vi "IVCurvePulsed.vi"(9 "Source Measure Unit Channel (0: Channel A)":i32, 10 "Waveform":waveform(dbl), 11 "VISA Refnum in":refnum<visa-resource-name>) -> (1 "appended array":dbl[][](array[numeric]), 3 "Cluster":cluster{"Y":dbl[], "Current (A)":dbl[]})   [LabVIEW 2020]
uses:
  <vilib>/Analysis/6fits.llb/Curve Fitting Criteria.ctl
  <vilib>/Utility/file.llb/Write Delimited Spreadsheet (DBL).vi
  Keithley 2600 Series/Keithley 2600 Series.lvlib
  <vilib>/Analysis/NI_AALPro.lvlib
panel:
  out "XY Graph 2":cluster{dbl[], dbl[]}[](graph)
  out "Fit":dbl[](array[numeric])
  out "error out 2":errorcluster
  out "Waveform Graph":waveform(dbl)(graph)
  out "XY Graph":T1(graph)
  out "error out":errorcluster
  in  "Source Code":string="-- The local functions are scoped at the project level, so that we can keep\n-- track of the reading buffers throughout the test.\nreset()\nsmua.reset()\nlocal systemNodes = {}\nlocal systemSmus = {}\nlocal systemSmuReadingBufferIndexes = {}\nlocal appendMode = 1\n\nlocal gOverrunDetected = false\n--==========================================================================\n-- This function tests for overruns in any of the system smus' trigger models.\n-- It returns an error to the application that will be displayed in a\n-- dialog box if an overrun occurs.\n--==========================================================================\nlocal _Overruncheck = function()\n    --==========================================================================\n    -- This function test the results of the value in the smu's trigger overrun\n    -- status register. -- It returns an error if an overrun occurs.\n    --\n    -- parameter   overrun     A bit pattern that contains the smu trigger overrun\n    --                         status register result\n    --==========================================================================\n    local TestOverrunBits = function(overrun, selNode, whichSmu)\n        local whichNode = [[localnode.]]\n        if (selNode.tsplink.node ~= localnode.tsplink.node) then\n            whichNode = [[node[]] .. selNode.tsplink.node .. [[].]]\n        end\n        whichNode = whichNode .. whichSmu .. [[ (]] .. selNode.model .. [[)]]\n        if (bit.test(overrun, 2)) then\n            gOverrunDetected = true\n            return(\"arm overrun on \" .. whichNode .. \"{eol}\")\n        elseif (bit.test(overrun, 3)) then\n            gOverrunDetected = true\n            return(\"source overrun on \" .. whichNode .. \"{eol}\")\n        elseif (bit.test(overrun, 4)) then\n            gOverrunDetected = true\n            return(\"measure overrun on \" .. whichNode .. \"{eol}\")\n        elseif (bit.test(overrun, 5)) then\n            gOverrunDetected = true\n        return(\"end pulse overrun on \" .. whichNode .. \"{eol}\")\n    else\n        return(\"\")\n    end\nend\n\n-- Report an overrun error only once.\nif(gOverrunDetected == false) then\n    local allSmusInOverrun = [[]]\n    \n    for i, selNode in ipairs(systemNodes) do\n        for j, selSmu in ipairs(systemSmus[i]) do\n            if(j == 1) then\n                local overrun = selNode.status.operation.instrument.smua.trigger_overrun.event\n                if (overrun > 0) then\n                    allSmusInOverrun = allSmusInOverrun .. TestOverrunBits(overrun, selNode, [[smua]])\n                end\n            elseif(j == 2) then\n                local overrun = selNode.status.operation.instrument.smub.trigger_overrun.event\n                if (overrun > 0) then\n                    allSmusInOverrun = allSmusInOverrun .. TestOverrunBits(overrun, selNode, [[smub]])\n                end\n            end\n        end\n    end\n    \n    if (gOverrunDetected == true) then\n        print(\"[{error}]Script stopped due to:{eol}\" .. allSmusInOverrun)\n    end\nend\nend\n\nlocal gComplianceDetected = false\n--==========================================================================\n-- Checks smus for voltage or current compliance.\n-- If a compliance event occurs, the message dialog box is presented to the\n-- user.\n--==========================================================================\nlocal _ComplianceCheck = function()\n    -- Report a compliance error only once.\n    if(gComplianceDetected == false) then\n        local allSmusInCompliance = [[]]\n        \n        for i, selNode in ipairs(systemNodes) do\n            for j, selSmu in ipairs(systemSmus[i]) do\n                local compDetect = selNode.status.measurement.instrument.event\n                if(compDetect > 0) then\n                    -- Compose and show error message\n                    local whichNode = [[localnode.]]\n                    if (selNode.tsplink.node ~= localnode.tsplink.node) then\n                        whichNode = [[node[]] .. selNode.tsplink.node .. [[].]]\n                    end\n                    local whichSmu = [[]]\n                    if(compDetect == 2) then\n                        whichSmu = whichNode .. [[smua]]\n                    elseif (compDetect == 4) then\n                        whichSmu = whichNode .. [[smub]]\n                    elseif (compDetect == 6) then\n                        whichSmu = whichNode .. [[smua and ]] .. whichNode .. [[smub]]\n                    end\n                    whichSmu = whichSmu .. [[ (]] .. selNode.model .. [[){eol}]]\n                    allSmusInCompliance = allSmusInCompliance .. whichSmu\n                    \n                    -- Set gComplianceDetected so we don't report the error again.\n                    gComplianceDetected = true\n                end\n            end\n        end\n        \n        if (gComplianceDetected == true) then\n            print(\"[{info}]Compliance detected on:{eol}\" .. allSmusInCompliance ..\n            \"{eol}Click the Advanced button and check the Source Limit setting.\")\n        end\n    end\nend\n\nlocal gTestAborted = false\n--==========================================================================\n-- This function waits up to a specified period for the sweeps to complete.\n-- If the delay parameter is -1, then the timeout is infinite. It returns true\n-- if all sweeping actions are complete. Otherwise, the return value is false.\n-- Note: If gTestAborted is true, this function returns false immediately.\n--\n-- parameter  interval     Maximum time to wait (in seconds).\n--==========================================================================\nlocal _WaitForComplete = function(interval)\n    local pollInterval = 0.1\n    \n    --==========================================================================\n    -- Checks the system smus for any that are still sweeping.\n    --==========================================================================\n    local IsSweepingComplete = function()\n        for i, selNode in ipairs(systemNodes) do\n            for j, selSmu in ipairs(systemSmus[i]) do\n                if (j == 1) then\n                    local statcond = selNode.status.operation.instrument.smua.condition\n                    if (bit.test(statcond,4)) then\n                        return false\n                    end\n                elseif (j == 2) then\n                    local statcond = selNode.status.operation.instrument.smub.condition\n                    if (bit.test(statcond,4)) then\n                        return false\n                    end\n                end\n            end\n        end\n        \n        return true\n    end\n    \n    local notimeout = false\n    if (interval < 0) then\n        notimeout = true\n        interval = 1\n    end\n    \n    while(interval > 0) do\n        -- Check the abort flag\n        if (gTestAborted == true) then\n            return false\n        end\n        \n        -- Check for errors\n        if (errorqueue.count > 0) then\n            return false\n        end\n        \n        -- Check for overruns and compliance\n        _Overruncheck()\n        _ComplianceCheck()\n        \n        if (IsSweepingComplete() == true) then\n            return true\n        end\n        \n        delay(pollInterval)\n        \n        if (notimeout == false) then\n            interval = interval - pollInterval\n        end\n    end\n    \n    if (IsSweepingComplete() == true) then\n        return true\n    end\n    \n    return false\nend\n----------------------------------------------------------------------------\n-- START OF INITIALIZE SEGMENT ... do not modify this section\n----------------------------------------------------------------------------\n--==========================================================================\n-- This function prepares the test for execution. \n-- It first verifies that current setup matches project's setup. \n-- Then, it initializes members used to keep track of reading buffer storage.\n--==========================================================================\nfunction _Initialize()\n    local maxNodes = 64   -- Maximum possible nodes in TSP link system.\n    \n    local projectSetup = {{localnode,[[2636A]],[[2.2.1]]}} -- Instrument configuration for the project.\n    local currentSetup = {} -- Current instrument configuration.\n    \n    local errorTag = \"[{error}]\"\n    local errorMessage = {[[Instrument in project configuration not found.]], [[Instrument configuration at does not match.]]}\n    local errorNo = 0\n    \n    --==========================================================================\n    -- Configures the status model to detect voltage or current compliance.\n    --==========================================================================\n    local ConfigStatusModel = function()\n        for i, selNode in ipairs(systemNodes) do\n            selNode.status.reset()\n            for j, selSmu in ipairs(systemSmus[i]) do\n                -- The selSmu.source.compliance call will force an update\n                -- the condition register of the measurement.instrument.smuX to\n                -- update\n                local dum = selSmu.source.compliance\n                if(j == 1) then\n                    -- Clear the measurement.instrument.smua event register by reading its value\n                    dum = selNode.status.measurement.instrument.smua.event\n                    -- Now configure the status model to detect voltage or current compliance\n                    selNode.status.measurement.instrument.smua.enable = 3\n                    selNode.status.measurement.instrument.smua.ptr = 3\n                    selNode.status.measurement.instrument.enable = 6\n                    selNode.status.measurement.instrument.ptr = 6\n                elseif(j == 2) then\n                    -- Clear the measurement.instrument.smub event register by reading its value\n                    dum = selNode.status.measurement.instrument.smub.event\n                    -- Now configure the status model to detect voltage or current compliance\n                    selNode.status.measurement.instrument.smub.enable = 3\n                    selNode.status.measurement.instrument.smub.ptr = 3\n                end\n            end\n        end\n    end\n    \n    --==========================================================================\n    -- Determines the current system configuration.\n    --==========================================================================\n    local GetSetup = function ()\n        local masterNode = tsplink.node\n        \n        systemSmus = {}\n        systemNodes = {}\n        systemNodes[1] = node[masterNode]\n        \n        currentSetup[1] = {}\n        currentSetup[1][1] = node[masterNode]\n        currentSetup[1][2] = node[masterNode].model\n        currentSetup[1][3] = node[masterNode].revision\n        \n        systemSmus[1] = {}\n        systemSmus[1][1] = node[masterNode].smua\n        \n        if(node[masterNode].smub ~= nil) then\n            systemSmus[1][2] = node[masterNode].smub\n        end\n        \n        local j = 2\n        for i = 1, maxNodes do\n            if((tsplink.node ~= i) and (node[i] ~= nil)) then\n                systemNodes[j] = node[i]\n                currentSetup[j] = {}\n                currentSetup[j][1] = node[i]\n                currentSetup[j][2] = node[i].model\n                currentSetup[j][3] = node[i].revision\n                \n                systemSmus[j] = {}\n                systemSmus[j][1] = node[i].smua\n                \n                if(node[i].smub ~= nil) then\n                    systemSmus[j][2] = node[i].smub\n                end\n                j = j +1\n            end\n        end\n    end\n    \n    GetSetup()\n    \n    -- Check the project setup versus the configuration setup.\n    -- If there is a difference, report an error.\n    local numpInstruments = table.getn(projectSetup)\n    local numcInstruments = table.getn(currentSetup)\n    \n    for i=1, numpInstruments do\n        local pfields = table.getn(projectSetup[i])\n        \n        errorNo = 1\n        for j=1,numcInstruments do\n            -- Compare nodes.\n            if(projectSetup[i][1] ==  currentSetup[j][1]) then\n                errorNo = 0\n                \n                for k=2, pfields do\n                    if(projectSetup[i][k] ~= currentSetup[j][k]) then\n                        errorNo = 2\n                    end\n                end\n                break\n            end\n        end\n        \n        if (errorNo > 0) then\n            break\n        end\n    end\n    \n    if (errorNo > 0) then\n        error(errorMessage[errorNo])\n        print(errorTag .. errorMessage[errorNo])\n    end\n    \n    --==========================================================================\n    -- Initializes all system readings buffers by clearing and setting them to\n    -- append mode. An array, sysSmuReadingBufferIndexes, is used to keep track of the\n    -- data stored to each of the reading buffers.\n    --==========================================================================\n    local InitalizeReadingBuffers = function()\n        systemSmuReadingBufferIndexes = {}\n        for i, selNode in ipairs(systemSmus) do\n            systemSmuReadingBufferIndexes[i] = {}\n            \n            for j, selSmu in ipairs(selNode) do\n                -- Create an array for the smu.\n                systemSmuReadingBufferIndexes[i][j] = {}\n                \n                local snvBuffers =  {selSmu.nvbuffer1, selSmu.nvbuffer2}\n                for k, selBuffer in ipairs(snvBuffers) do\n                    -- Create an array for nvbuffers 1 and 2.\n                    systemSmuReadingBufferIndexes[i][j][k] = {}\n                    \n                    local sysSmuReadingBufferIndexes = systemSmuReadingBufferIndexes[i][j][k]\n                    sysSmuReadingBufferIndexes[\"start\"] = 0\n                    sysSmuReadingBufferIndexes[\"stop\"] = 0\n                    \n                    selBuffer.clear()\n                    selBuffer.appendmode = 1\n                    selBuffer.collecttimestamps = 1\n                    selBuffer.collectsourcevalues = 1\n                    selBuffer.timestampresolution = 1e-6\n                    if (selBuffer.fillmode ~= nil) then\n                        selBuffer.fillmode = selSmu.FILL_ONCE\n                    end\n                end\n                \n            end\n        end\n    end\n    \n    InitalizeReadingBuffers()\n    ConfigStatusModel()\nend\n----------------------------------------------------------------------------\n-- END OF INITIALIZE SEGMENT ... do not modify code after this point\n----------------------------------------------------------------------------\n\n----------------------------------------------------------------------------\n-- START OF SWEEP SEGMENT ... do not modify this section\n----------------------------------------------------------------------------\n--==========================================================================\n-- Configures a sweeping test.\n-- (This represents a Sweep segment of the script.  Click on the Sweep tab to customize it.)\n--==========================================================================\nfunction _Sweep()\n    local highSpeedSampling = false\n    local errorTag = \"[{error}]\"\n    local biasIndex = 1\n    local stepIndex = 2\n    local sweepIndex = 3\n    local numLevels = 3\n    local nvBuffersUsed = {1,1,1}\n    -- local alias for SMUs\n    local sweep1 = localnode.smua -- is a 2636A\n    -- \"NoStepFixed\" configuration (autorange enabled = false,  #step channels = 0):\n    -- This function configures any number of sweeping smus with no stepping smus.\n    -- It supports sweeps with autorange off and pulse mode.\n    local testSmus = {\n        {{}},  -- Bias\n        {{}},  -- Step\n        {{ localnode.smua }},  -- Sweep\n    }\n    \n    local testNodes = {\n        {},  -- Bias\n        {},  -- Step\n        {localnode}  -- Sweep\n    }\n    \n    local sweepPulseModes ={{ false }}\n    \n    local timePoint = 0.1\n    local pulseWidth = 99.0000009537E-3\n    local measurePointTime = 16.7266666667E-3\n    \n    local numberOfSteps  =  1\n    local numberOfSweeps = #NumPoints\n    \n    local nplc = 1\n    local lineFrequency = 60\n    \n    local numNodes = table.getn(testNodes[sweepIndex])\n    local numMasterSmus = table.getn(testSmus[sweepIndex][1])\n    local masterNode = testNodes[sweepIndex][1]\n    local masterSweepSmu = testSmus[sweepIndex][1][1]\n    \n    local t1Timer = masterNode.trigger.timer[1]    -- t1Timer is for sweep time per point\n    local t2Timer = masterNode.trigger.timer[2]    -- t2Timer is for sweep pulse width\n    local t3Timer = masterNode.trigger.timer[3]    -- t3Timer is for a 1ms initial delay\n    \n    local masterTspLine1 = masterNode.tsplink.trigger[1]    -- for source stimulus\n    local masterTspLine2 = masterNode.tsplink.trigger[2]    -- for endpulse stimulus\n    \n    --==========================================================================\n    -- This function checks for errors or conflicts in the test settings (timing, ranges, etc.)\n    --==========================================================================\n    local CheckSettings = function()\n        local measureDelay = timePoint - measurePointTime\n        \n        local errorMsg = nil\n        \n        -- Valid timing paramaters\n        -- None of these errors should appear to the user.\n        if (masterSweepSmu == nil) then\n            errorMsg =  [[Must have at least one sweeping smu.]]\n        elseif (timePoint <= 0) then\n            errorMsg = [[timePoint <= 0]]\n        elseif (pulseWidth <= 0) then\n            errorMsg = [[pulseWidth <= 0]]\n        elseif (pulseWidth > timePoint) then\n            errorMsg = [[pulseWidth > timePoint]]\n        elseif (measureDelay < 0) then\n            errorMsg = [[timePoint too small, <= measurePointTime]]\n        end\n        \n        if (errorMsg ~= nil) then\n            print(errorTag.. errorMsg)\n            error(errorMsg)\n        end\n    end\n    \n    --==========================================================================\n    -- This function configures the trigger line interaction between the smus.\n    --==========================================================================\n    local ConfigureTriggerLines = function()\n        --==========================================================================\n        -- This function configures the timers that are used in the test.\n        --==========================================================================\n        local ConfigureSweepTimers = function()\n            -- t3Timer provides a 1ms initial delay following the masterSweepSmu's armed event ID.\n            -- This is to ensure that masterSweepSmu is fully ready for the first source stimulus.\n            t3Timer.stimulus = masterSweepSmu.trigger.ARMED_EVENT_ID\n            t3Timer.passthrough = false\n            t3Timer.delay = 1.0e-3\n            t3Timer.count = 1\n            \n            if (numberOfSweeps > 1) then\n                t1Timer.stimulus = t3Timer.EVENT_ID\n                t1Timer.passthrough = true\n                t1Timer.delay = timePoint\n                t1Timer.count = numberOfSweeps - 1\n                \n                t2Timer.stimulus = t1Timer.EVENT_ID\n            else\n                -- Cannot use t1Timer when numberOfSweeps <= 1\n                t2Timer.stimulus = t3Timer.EVENT_ID\n            end\n            \n            t2Timer.passthrough = false\n            t2Timer.delay = pulseWidth\n            t2Timer.count = 1\n        end\n        \n        --==========================================================================\n        -- This function configures the sweeping smus.\n        --==========================================================================\n        local ConfigureSweep = function()\n            \n            --==========================================================================\n            -- This function configures all sweeping smus on the master node.\n            --==========================================================================\n            local ConfigureMasterNodeSweepSmus = function()\n                for i=1, numMasterSmus do\n                    local pulseMode = sweepPulseModes[1][i]\n                    local selSmu = testSmus[sweepIndex][1][i]\n                    local sourceStimulus = masterTspLine1.EVENT_ID\n                    \n                    if (i==1) then\n                        -- masterSweepSmu will be triggered by StartSweep()\n                        -- Use a dummy event ID as a place holder for the arm stimulus\n                        selSmu.trigger.arm.stimulus = masterNode.trigger.EVENT_ID\n                    else\n                        selSmu.trigger.arm.stimulus = 0\n                    end\n                    \n                    selSmu.trigger.source.stimulus = sourceStimulus\n                    selSmu.trigger.source.action = selSmu.ENABLE\n                    \n                    if ((pulseMode == true) and (pulseWidth < timePoint)) then\n                        selSmu.trigger.endpulse.stimulus = masterTspLine2.EVENT_ID\n                        selSmu.trigger.endpulse.action = selSmu.SOURCE_IDLE\n                    else\n                        selSmu.trigger.endpulse.stimulus = selSmu.trigger.MEASURE_COMPLETE_EVENT_ID\n                        selSmu.trigger.endpulse.action = selSmu.SOURCE_HOLD\n                    end\n                    \n                    if (highSpeedSampling == true) then\n                        selSmu.trigger.measure.stimulus = sourceStimulus\n                        selSmu.trigger.measure.action = selSmu.ASYNC\n                        \n                        -- Cannot collect source values when in asynchronous mode\n                        selSmu.nvbuffer1.collectsourcevalues = 0\n                        selSmu.nvbuffer2.collectsourcevalues = 0\n                    else\n                        selSmu.trigger.measure.stimulus = 0\n                        selSmu.trigger.measure.action = selSmu.ENABLE\n                    end\n                    \n                    selSmu.trigger.arm.count = numberOfSteps\n                    selSmu.trigger.count = numberOfSweeps\n                end\n            end\n            \n            --==========================================================================\n            -- This function configures a sweeping smu on a remote node\n            --\n            -- parameter pulseMode      true for Pulse mode,  false otherwise.\n            -- parameter selNode        Node to which the smu belongs.\n            -- parameter selSmu         Smu to configure.\n            --==========================================================================\n            local ConfigureRemoteSweepSmu = function(pulseMode, selNode, selSmu)\n                local tspl1 = selNode.tsplink.trigger[1]\n                local tspl2 = selNode.tsplink.trigger[2]\n                local sourceStimulus = tspl1.EVENT_ID\n                \n                selSmu.trigger.arm.stimulus = 0\n                selSmu.trigger.source.stimulus = sourceStimulus\n                selSmu.trigger.source.action = selSmu.ENABLE\n                \n                if ((pulseMode == true) and (pulseWidth < timePoint)) then\n                    selSmu.trigger.endpulse.stimulus = tspl2.EVENT_ID\n                    selSmu.trigger.endpulse.action = selSmu.SOURCE_IDLE\n                else\n                    selSmu.trigger.endpulse.stimulus = selSmu.trigger.MEASURE_COMPLETE_EVENT_ID\n                    selSmu.trigger.endpulse.action = selSmu.SOURCE_HOLD\n                end\n                \n                if (highSpeedSampling == true) then\n                    selSmu.trigger.measure.stimulus = sourceStimulus\n                    selSmu.trigger.measure.action = selSmu.ASYNC\n                    \n                    -- Cannot collect source values when in asynchronous mode\n                    selSmu.nvbuffer1.collectsourcevalues = 0\n                    selSmu.nvbuffer2.collectsourcevalues = 0\n                else\n                    selSmu.trigger.measure.stimulus = 0\n                    selSmu.trigger.measure.action = selSmu.ENABLE\n                end\n                \n                selSmu.trigger.arm.count = numberOfSteps\n                selSmu.trigger.count = numberOfSweeps\n            end\n            \n            --===========================\n            -- START of ConfigureSweep()\n            --===========================\n            -- Prepare a tsplink trigger line for source stimulus on the master node\n            masterTspLine1.mode = tsplink.TRIG_FALLING\n            masterTspLine1.pulsewidth = 1e-6\n            if (numberOfSweeps > 1) then\n                masterTspLine1.stimulus = t1Timer.EVENT_ID\n            else\n                masterTspLine1.stimulus = t3Timer.EVENT_ID\n            end\n            \n            -- Prepare a tsplink trigger line for endpulse stimulus on the master node\n            masterTspLine2.mode = tsplink.TRIG_FALLING\n            masterTspLine2.pulsewidth = 1e-6\n            masterTspLine2.stimulus = t2Timer.EVENT_ID\n            \n            -- Configure all sweep smus on the master node.\n            -- The master node contains the smu that kicks off the sweeps.\n            ConfigureMasterNodeSweepSmus()\n            \n            -- Configure the sweeping smus on remote nodes\n            if (numNodes > 1) then\n                for i=2, numNodes do\n                    -- For each remote node, configure the tsplink trigger lines\n                    local selNode = testNodes[sweepIndex][i]\n                    \n                    local tspl1 = selNode.tsplink.trigger[1]\n                    tspl1.mode = tsplink.TRIG_FALLING\n                    tspl1.pulsewidth = 1e-6\n                    tspl1.stimulus = 0\n                    \n                    local tspl2 = selNode.tsplink.trigger[2]\n                    tspl2.mode = tsplink.TRIG_FALLING\n                    tspl2.pulsewidth = 1e-6\n                    tspl2.stimulus = 0\n                    \n                    local sweepSmus = testSmus[sweepIndex]\n                    local numSmus = table.getn(sweepSmus[i])\n                    \n                    for j=1, numSmus do\n                        -- For each sweeping smu on each remote node, configure the remote sweeping smu\n                        local extSmu  = sweepSmus[i][j]\n                        local pulseMode = sweepPulseModes[i][j]\n                        \n                        ConfigureRemoteSweepSmu(pulseMode, selNode, extSmu)\n                    end\n                end\n            end\n        end\n        \n        -- Configure timers and sweep trigger lines.\n        ConfigureSweepTimers()\n        ConfigureSweep()\n    end\n    \n    --==========================================================================\n    -- This function kicks off the sweep.\n    --==========================================================================\n    local StartSweep = function()\n        masterSweepSmu.trigger.arm.set()\n    end\n    --==========================================================================\n    -- Resets all components that may be used in the test.\n    --==========================================================================\n    local Reset = function()\n        for i, selTest in ipairs(testSmus) do\n            for j, selNode in ipairs(testNodes[i]) do\n                if(selNode ~= nil) then\n                    -- Reset blenders\n                    local k = 1\n                    while(selNode.tsplink.trigger[k] ~= nil) do\n                        selNode.tsplink.trigger[k].reset()\n                        k = k+1\n                    end\n                    \n                    k=1\n                    while(selNode.trigger.blender[k] ~= nil) do\n                        selNode.trigger.blender[k].reset()\n                        k = k+1\n                    end\n                    \n                    -- Reset Timers\n                    k =1\n                    while(selNode.trigger.timer[k] ~= nil) do\n                        selNode.trigger.timer[k].reset()\n                        k = k+1\n                    end\n                end\n            end\n            \n            -- Reset Smus\n            for j, selNode in ipairs(selTest) do\n                for k, selSmu in ipairs(selNode) do\n                    if(selSmu ~= nil) then\n                        -- Resets all smus in the test.\n                        selSmu.reset()\n                    end\n                end\n            end\n        end\n    end\n    \n    --==========================================================================\n    -- Turns all smus in the test on.\n    --==========================================================================\n    local TurnSmusOn = function()\n        for i, selTest in ipairs(testSmus) do\n            for j, selNode in ipairs(selTest) do\n                for k, selSmu in ipairs(selNode) do\n                    if(selSmu ~= nil) then\n                        if(selSmu.source.output ~= 1) then\n                            selSmu.source.output = 1\n                        end\n                    end\n                end\n            end\n        end\n    end\n    \n    --==========================================================================\n    -- This function initiates the steping and sweeping smus.\n    --==========================================================================\n    local InitiateSmus = function()\n        for i=2,numLevels do\n            for j, selNode in ipairs(testSmus[i]) do\n                for k, selSmu in ipairs(selNode) do\n                    if(selSmu ~= nil) then\n                        selSmu.trigger.initiate()\n                    end\n                end\n            end\n        end\n    end\n    \n    --==========================================================================\n    -- This function determines the number of points that will be in the buffer at the end of the test.\n    --==========================================================================\n    local StoreReadingBufferIndexes = function()\n        --==========================================================================\n        -- Determines reading buffer starting and stopping indexes.\n        -- parameter    testLevel    Index referring to bias, step, or sweep.\n        -- parameter    i            Node index.\n        -- parameter    selSmuIndex  Selected smu index.\n        --==========================================================================\n        local SetupLastPoints = function(testLevel, i, selSmuIndex)\n            local stoppingPoint1 = 0\n            local stoppingPoint2 = 0\n            local incVal = 0\n            local selSmuRbIndex1 = systemSmuReadingBufferIndexes[i][selSmuIndex][1]\n            local selSmuRbIndex2 = systemSmuReadingBufferIndexes[i][selSmuIndex][2]\n            \n            selSmuRbIndex1[\"start\"] = 1\n            selSmuRbIndex2[\"start\"] = 1\n            \n            -- appendMode is a local variable common to the script.\n            if(appendMode == 1) then\n                stoppingPoint1 = selSmuRbIndex1[\"stop\"]\n                stoppingPoint2 = selSmuRbIndex2[\"stop\"]\n            end\n            -- Bias setup\n            if(testLevel == biasIndex) then\n                incVal = 1\n                -- Step setup\n            elseif (testLevel == stepIndex) then\n                incVal = (1 * 1)\n                -- Sweep setup\n            elseif (testLevel == sweepIndex) then\n                if (highSpeedSampling == true) then\n                    incVal = (1 * 200 * 60)\n                else\n                    incVal = (1 * 200 * 1)\n                end\n            end\n            \n            selSmuRbIndex1[\"stop\"] = stoppingPoint1 + incVal\n            if(nvBuffersUsed[testLevel] == 2) then\n                selSmuRbIndex2[\"stop\"] = stoppingPoint2 + incVal\n            end\n        end\n        \n        for i, selTest in ipairs(testSmus) do\n            for j, selNode in ipairs(selTest) do\n                for k, selSmu in ipairs(selNode) do\n                    for l, selSysNode in ipairs(systemSmus) do\n                        if(selSysNode[1] == selSmu) then\n                            SetupLastPoints(i, l, 1)\n                        end\n                        \n                        if(selSysNode[2] ~= nil) then\n                            if(selSysNode[2] == selSmu) then\n                                SetupLastPoints(i, l, 2)\n                            end\n                        end\n                    end\n                end\n            end\n        end\n    end\n    ---==========================================================================\n    -- The following makes sure we capture a measurement from the bias channels\n    --==========================================================================\n    local MeasureBiasChannels = function()\n    end\n    --==========================================================================\n    -- This function Configures the smu options such as nplc, function, range, etc.\n    --==========================================================================\n    local ConfigureSmus = function()\n        -- set up Sweep (inner sweep) for sweep1\n        sweep1.sense = sweep1.SENSE_LOCAL\n        sweep1.source.delay = 0\n        sweep1.measure.nplc = nplc\n        sweep1.measure.autozero = sweep1.AUTOZERO_OFF\n        sweep1.measure.count = 1\n        sweep1.measure.filter.enable = sweep1.FILTER_OFF\n        sweep1.measure.filter.type = sweep1.FILTER_MOVING_AVG\n        sweep1.measure.filter.count = 1\n        sweep1.measure.delay = 0\n        sweep1.measure.delayfactor = 1\n        sweep1.measure.analogfilter = 0\n        sweep1.source.func = sweep1.OUTPUT_DCVOLTS\n        if sweep1.source.highc == sweep1.ENABLE then sweep1.source.highc = sweep1.DISABLE end\n        sweep1.source.limiti = 10E-3\n        sweep1.trigger.source.limiti = sweep1.LIMIT_AUTO\n        sweep1.source.autorangev = 0\n        sweep1.source.rangev = 2\n        sweep1.trigger.source.listv({#VoltList})\n        sweep1.measure.autorangei = 0\n        sweep1.measure.rangei = 100E-12\n        sweep1.measure.autorangev = sweep1.source.autorangev\n        if (sweep1.measure.autorangev == 0) then\n            sweep1.measure.rangev = sweep1.source.rangev\n        end\n        sweep1.trigger.measure.iv(sweep1.nvbuffer1, sweep1.nvbuffer2)\n        nvBuffersUsed[sweepIndex] = 2\n    end\n    -- Test starts here.\n    \n    -- Make sure previous test is done.\n    \n    _WaitForComplete(-1)\n    \n    CheckSettings()\n    Reset()\n    ConfigureSmus()\n    ConfigureTriggerLines()\n    \n    StoreReadingBufferIndexes()\n    TurnSmusOn()\n    MeasureBiasChannels()\nsmua.source.levelv = 0\n\n    InitiateSmus()\n     delay(1)\n    StartSweep()\nend\n----------------------------------------------------------------------------\n-- END OF SWEEP SEGMENT ... do not modify code after this point\n----------------------------------------------------------------------------\n\n----------------------------------------------------------------------------\n-- START OF DATAREPORT SEGMENT ... do not modify this section\n----------------------------------------------------------------------------\n--==========================================================================\n-- This script returns a series of reading buffers. \n-- (This represents a DataReport segment of the script.  Click on the Data tab to customize it.)\n--==========================================================================\nfunction _Data()\n    local buffers = {localnode.smua.nvbuffer1,localnode.smua.nvbuffer2} -- Array of reading buffers to return\n    local bufferNames = {[[localnode.smua.nvbuffer1]],[[localnode.smua.nvbuffer2]]} -- Array of reading buffer names\n    local bufferSmuNames = {[[Sweep_SMU]],[[Sweep_SMU]]} -- Array of SMU names for each reading buffer\n    local expectedCount = {} -- Array containing the expected number of return values.\n    local waitInterval = 1  -- Interval between message transfers\n    local maxToReturn = 100 -- Maximum reading buffer points between message transfers.\n    \n    -- The following are special tokens used internally by the data report function\n    local DATA_REPORT = \"(({{Data}}))\"\n    local SWEEPSTART = \"{SWEEP-START}\"\n    local START = \"{START}\"\n    local NAME = \"{NAME}\"\n    local EXPECTED_COUNT = \"{EXPECTED-COUNT}\"\n    local PTS_IN_BUFF = \"{PTS-IN-BUFF}\"\n    local PTS_RETURNED =  \"{PTS-RETURNED}\"\n    local BASE_TIME_STAMP = \"{BASE-TIME-STAMP}\"\n    local READINGS = \"{READINGS}\"\n    local TIMESTAMPS = \"{TIMESTAMPS}\"\n    local SRCVALS = \"{SRCVALS}\"\n    local END = \"{END}\"\n    local COMPLETE = \"{COMPLETE}\"\n    \n    local errorTag = \"[{error}]\"\n    local dataIndexes = {} -- Data transfer index for each reading buffer\n    local done = true  -- True when data transfer from all of reading buffers is completed\n    local dataComplete = true  -- True when all of reading buffers have reached their expected counts\n    \n    --==========================================================================\n    -- This function determines the ending points that will be in the buffer\n    -- at the time data collection takes place.\n    --==========================================================================\n    local GetStopPoints = function()\n        for i, selBuffer in ipairs(buffers) do\n            for j, selSysNode in ipairs(systemSmus) do\n                for k, selSmu in ipairs(selSysNode) do\n                    if (selSmu.nvbuffer1 == selBuffer) then\n                        expectedCount[i] = systemSmuReadingBufferIndexes[j][k][1][\"stop\"]\n                    elseif (selSmu.nvbuffer2 == selBuffer) then\n                        expectedCount[i] = systemSmuReadingBufferIndexes[j][k][2][\"stop\"]\n                    end\n                end\n            end\n        end\n    end\n    \n    --==========================================================================\n    -- Checks if the SMU for selBuffer is sweeping.\n    --==========================================================================\n    local IsSweeping = function(selBuffer)\n        for i, selNode in ipairs(systemNodes) do\n            for j, selSmu in ipairs(systemSmus[i]) do\n                if (j == 1) then\n                    if ((selSmu.nvbuffer1 == selBuffer) or (selSmu.nvbuffer2 == selBuffer)) then\n                        local statcond = selNode.status.operation.instrument.smua.condition\n                        return (bit.test(statcond,4))  -- Check Bit B3, Sweeping (SWE)\n                    end\n                elseif (j == 2) then\n                    if ((selSmu.nvbuffer1 == selBuffer) or (selSmu.nvbuffer2 == selBuffer)) then\n                        local statcond = selNode.status.operation.instrument.smub.condition\n                        return (bit.test(statcond,4))  -- Check Bit B3, Sweeping (SWE)\n                    end\n                end\n            end\n        end\n        return false\n    end\n    \n    --==========================================================================\n    -- Clears the reading buffers and resets the array that contains the\n    -- reading buffer storage start/ stop points.\n    --==========================================================================\n    local ClearReturnedBuffers = function()\n        for i, selBuffer in ipairs(buffers) do\n            selBuffer.clear()\n            \n            local smuBufferIndex = nil\n            for j, selSysNode in ipairs(systemSmus) do\n                for k, selSmu in ipairs(selSysNode) do\n                    if (selSmu.nvbuffer1 == selBuffer) then\n                        smuBufferIndex = systemSmuReadingBufferIndexes[j][k][1]\n                    elseif (selSmu.nvbuffer2 == selBuffer) then\n                        smuBufferIndex = systemSmuReadingBufferIndexes[j][k][2]\n                    end\n                end\n            end\n            if(smuBufferIndex ~= nil) then\n                smuBufferIndex[\"start\"] = 0\n                smuBufferIndex[\"stop\"] = 0\n            end\n        end\n    end\n    \n    GetStopPoints()\n    \n    -- Initialize dataIndex. This array is used to keep track of the points returned to\n    -- the application.\n    \n    for i, v in ipairs(buffers) do\n        dataIndexes[i] = 1\n    end\n    \n    -- The following print statements turns on data report feature within the application.\n\n    \n    repeat\n        done = true\n        dataComplete = true\n        for i, selBuffer in ipairs(buffers) do\n            -- Check for smu trigger model overruns.\n            _Overruncheck()\n            \n            -- Check for smu compliance.\n            _ComplianceCheck()\n            \n            -- Caution: Check for stillSweeping BEFORE getting numPointsStored\n            local stillSweeping = IsSweeping(selBuffer)\n            local numPointsStored = selBuffer.n\n            \n            -- Check for sweep completion before data is complete (i.e. something bad happened)\n            if ((numPointsStored < expectedCount[i]) and (stillSweeping == false)) then\n                gTestAborted = true\n            end\n            \n            dataComplete = dataComplete and (numPointsStored >= expectedCount[i])\n            done = done and (dataIndexes[i] > expectedCount[i])\n            \n            if(dataIndexes[i] <= numPointsStored) then\n                local points = numPointsStored - dataIndexes[i] + 1\n                \n                if(points > maxToReturn) then\n                    points = maxToReturn\n                end\n                \n                local retString = string.format(\"%d,%d,\", i,  points )\n                \n                               \n                local start = dataIndexes[i]\n                local stop = start + points -1\n                \n                local readings =\"\"\n                \n                for j=start, stop do\n                    if(j == start) then\n                        readings = readings .. string.format(\"%e,\",  selBuffer.readings[j])\n                    else\n                        readings = readings .. string.format(\"%e,\", selBuffer.readings[j])\n                    end\n                end\n                \n                local timestamps = \"\"\n                if (selBuffer.collecttimestamps == 1) then\n                    for j=start, stop do\n                        if(j == start) then\n                            timestamps = timestamps .. string.format(\"%e,\", selBuffer.timestamps[j])\n                        else\n                            timestamps = timestamps .. string.format(\"%e,\", selBuffer.timestamps[j])\n                        end\n                    end\n                end\n                \n                local srcValues = \"\"\n                if (selBuffer.collectsourcevalues == 1) then\n                    for j=start, stop do\n                        if(j == start) then\n                            srcValues = srcValues .. string.format(\"%e,\",  selBuffer.sourcevalues[j])\n                        else\n                            srcValues = srcValues .. string.format(\"%e,\", selBuffer.sourcevalues[j])\n                        end\n                    end\n                end\n                \n                dataIndexes[i] = stop +1\n                \n               \n                print(string.format(\"%d,%d,\", i+1,  points ) .. readings )\n                print(string.format(\"%d,%d,\", 0,  points ) .. timestamps)\n                print(string.format(\"%d,%d,\", 1,  points ) .. srcValues)\n\n            end\n        end\n        \n        if(dataComplete == false) then\n            if (gTestAborted == true) then\n                done = true  -- Stop waiting for data completion because it will never happen\n            else\n                delay(waitInterval)\n            end\n        end\n    until (done == true)\n    \n    print(COMPLETE .. \"\\n\")\n    \n    -- The application may not have selected all the buffers being used in the test, so\n    -- we need to make sure the overlapped operations are complete before clearing the buffers.\n    local sweepCompleted = _WaitForComplete(-1)\n    \n    if (sweepCompleted == true) then\n        ClearReturnedBuffers()\n    end\nend\n----------------------------------------------------------------------------\n-- END OF DATAREPORT SEGMENT ... do not modify code after this point\n----------------------------------------------------------------------------\n\n----------------------------------------------------------------------------\n-- START OF FINALIZE SEGMENT ... do not modify this section\n----------------------------------------------------------------------------\n--==========================================================================\n-- The function completes the script and places the instrument in a known state.\n--==========================================================================\nfunction _Finalize()\n    -- Wait for test completion\n    local sweepCompleted = _WaitForComplete(-1)\n    \n    -- Check for abnornal completion\n    if (sweepCompleted == false) then\n        -- Abort all overlapped operations on all smus\n        for i, selNode in ipairs(systemNodes) do\n            for j, selSmu in ipairs(systemSmus[i]) do\n                selSmu.abort()\n            end\n        end\n        \n        -- Check for errors\n        if (errorqueue.count > 0) then\n            print(\"[{error}]Script stopped due to error(s).\" )\n        else\n            print(\"[{error}]Script stopped before completion.\" )\n        end\n    end\n    \n    -- Set output level to 0V and 0A for all SMUs\n    for i, selNode in ipairs(systemNodes) do\n        for j, selSmu in ipairs(systemSmus[i]) do\n            selSmu.source.leveli = 0\n            selSmu.source.levelv = 0\n        end\n    end\n    \n    -- Turn output off for all SMUs\n    for i, selNode in ipairs(systemNodes) do\n        for j, selSmu in ipairs(systemSmus[i]) do\n            selSmu.source.output = 0\n        end\n    end\n    \n    -- Reset the system,  placing it into a known safe state.\n    reset()\nend\n----------------------------------------------------------------------------\n-- END OF FINALIZE SEGMENT ... do not modify code after this point\n----------------------------------------------------------------------------\n\n_Initialize()\n_Sweep()\n_Data()\n_Finalize()\n\n"
  in  "Script Variable (myScript)":string="myScript"
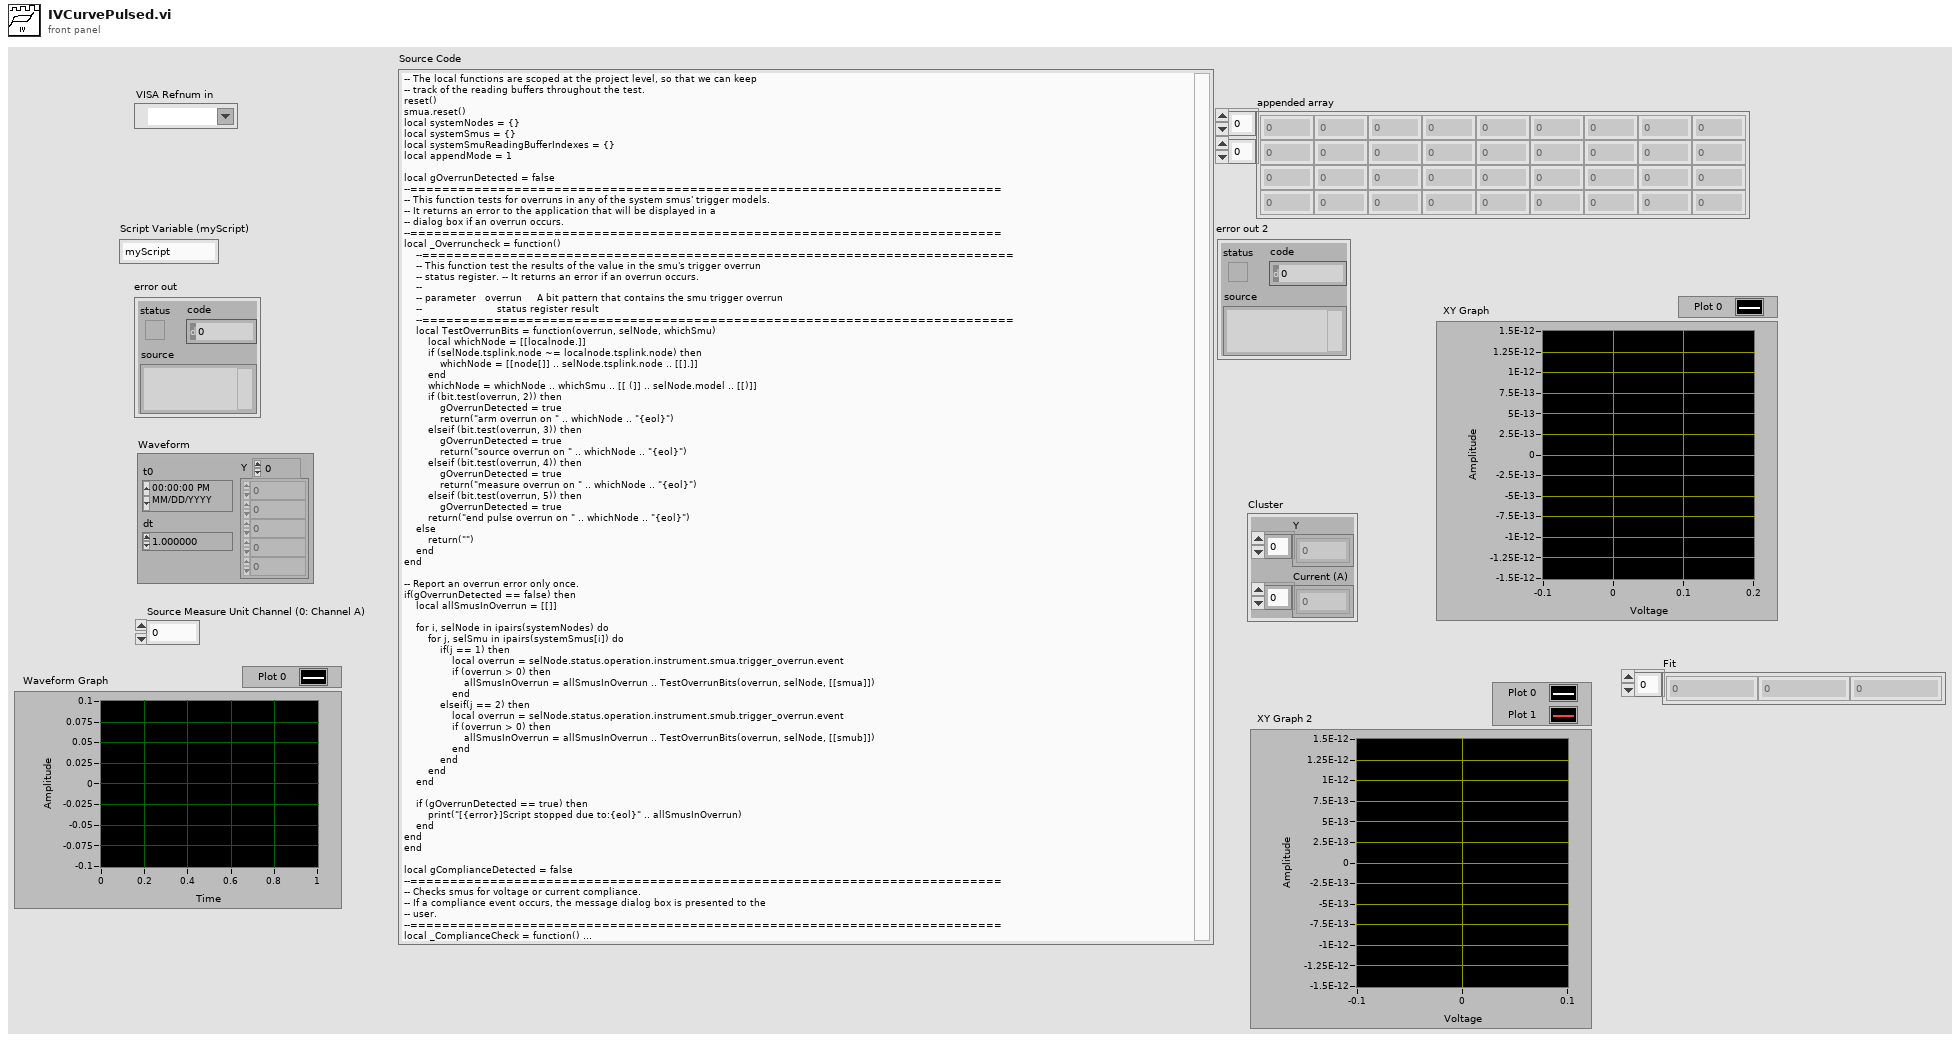
[diagram p1: front panel]
types:
  T1 = cluster{"array type (2D Dbl)":dbl[], "array type (2D Dbl)":dbl[]}
  T2 = typedef "NI_AALPro.lvlib/Curve Fitting Criteria.ctl" = u16
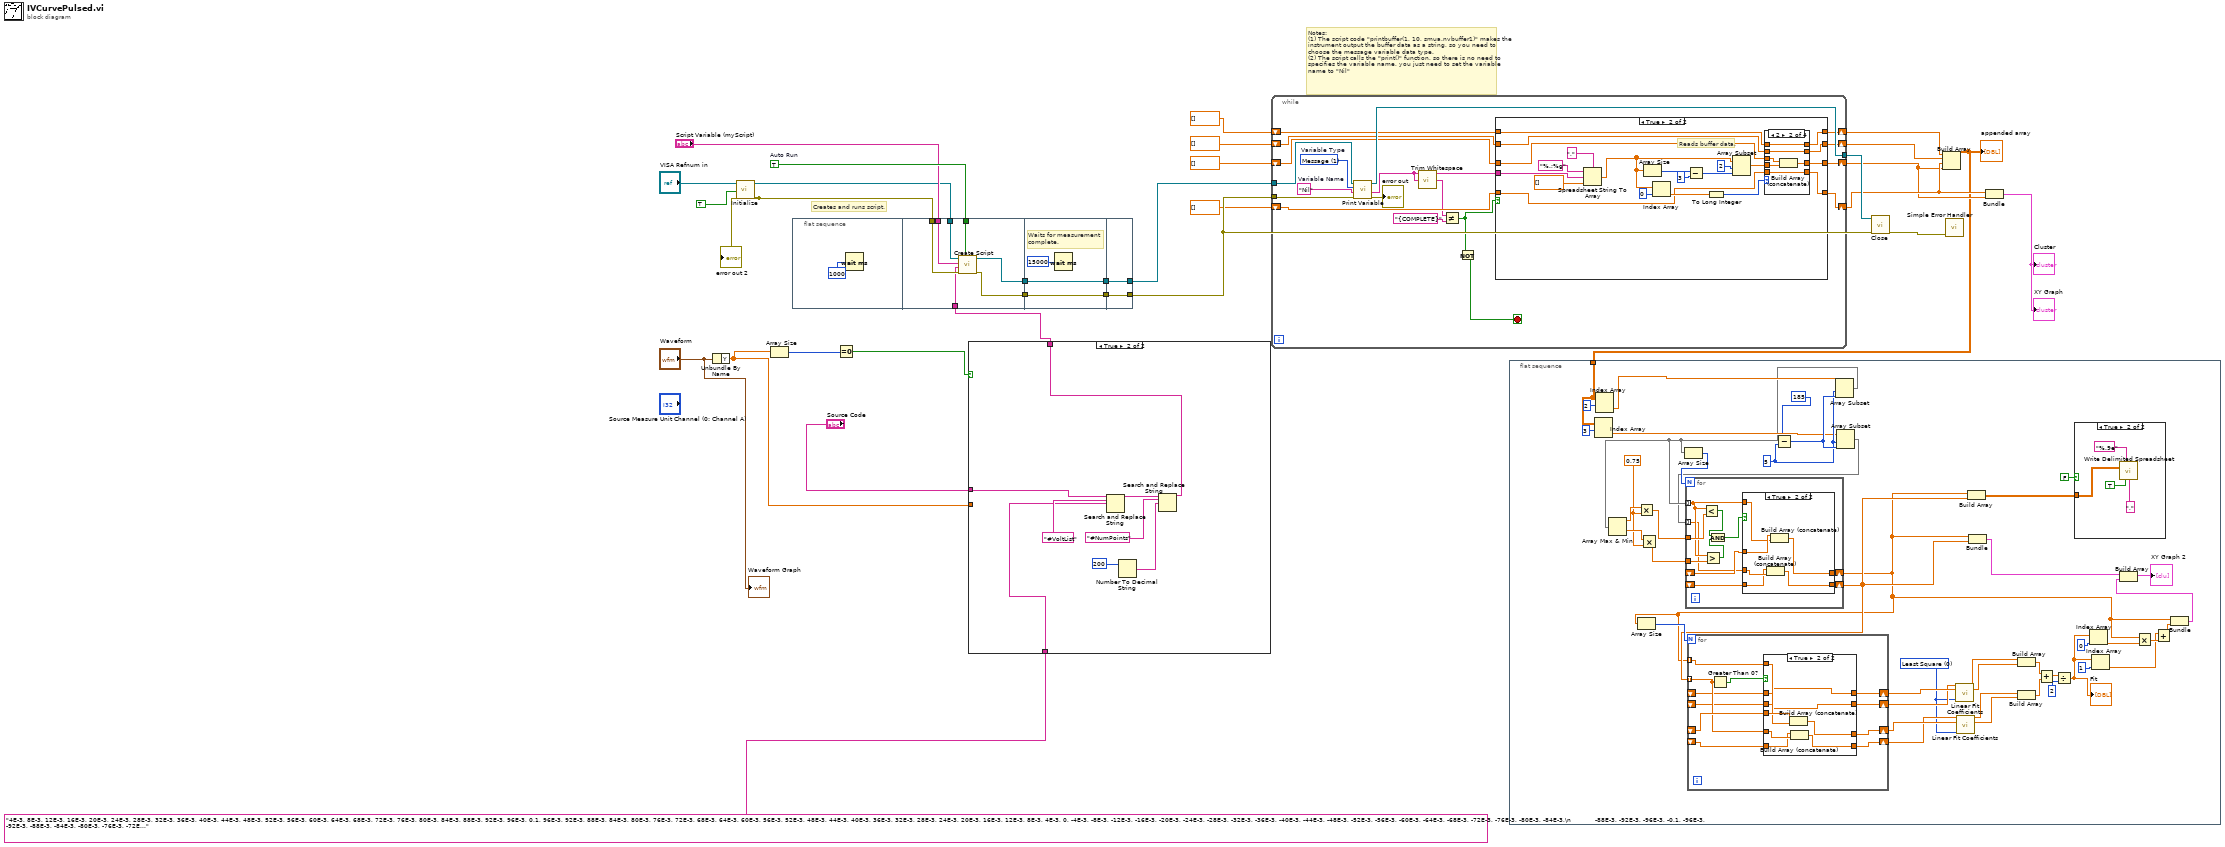
[diagram p0: block diagram]
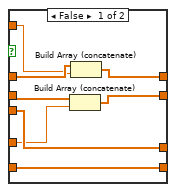
[diagram p2: hidden frame]
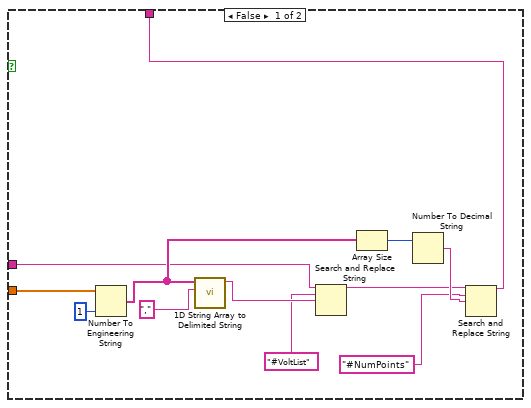
[diagram p5: hidden frame]
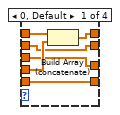
[diagram p7: hidden frame]
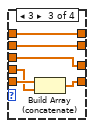
[diagram p8: hidden frame]
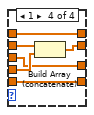
[diagram p9: hidden frame]
diagram:
  w16 = TRUE  # Auto Run
  # "Notes: \n(1) The script code \"printbuffer(1, 10, smua.nvbuffer1)\" makes the instrument output the buffer data as a string, so you need to choose the message variable data type.\n(2) The script calls the \"print()\" function, so there is no need to specifies the variable name, you just need to set the variable name to \"Nil\""
  # "Creates and runs script."
  n1 = Unbundle By Name("Waveform") -> ("Y"=w5:dbl[])
  n2 = call "Initialize.vi"("Reset (True)"=TRUE, "VISA resource name"="VISA Refnum in") -> ("error out"=w15:errorcluster, "VISA resource name out"=w13:refnum<visa-resource-name>)  [unwired: 8 in]
  "error out 2" <- w15
  n3 = Array Size(array=w5) -> (size(s)=w11:i32)
  n4 = flat-sequence {
    tunnel: [w34] -> w20
    tunnel: [w33] -> w19
    tunnel: w16 -> [w39]
    tunnel: w15 -> [w38]
    tunnel: w8 -> [w37]
    tunnel: "Script Variable (myScript)" -> [w36]
    tunnel: w13 -> [w35]
    tunnel: w20 -> [w42]
    tunnel: w19 -> [w41]
    tunnel: [w42] -> w18
    tunnel: [w41] -> w17
    tunnel: [w43] -> w29
    tunnel: [w44] -> w30
    tunnel: w18 -> [w44]
    tunnel: w17 -> [w43]
    frame #0 {
      n5 = Wait (ms)(milliseconds to wait=u32 1000) -> ()  [unwired: 1 out]
    }
    frame #1 {
      n6 = call "Create Script.vi"("Auto Run (F: Disable)"=w39, "error in (no error)"=w38, "Source Code"=w37, "Script Variable"=w36, "VISA resource name"=w35) -> ("error out"=w34:errorcluster, "VISA resource name out"=w33:refnum<visa-resource-name>)  [unwired: 5 in]
    }
    frame #2 {
      # "Waits for measurement complete."
      n7 = Wait (ms)(milliseconds to wait=15000) -> ()  [unwired: 1 out]
    }
    frame #3 {
    }
  }
  n8 = Equal To 0?(x=w11) -> (x = 0?=w10:bool)
  n9 = case shown="True" w10 {
    tunnel: "4E-3, 8E-3, 12E-3, 16E-3, 20E-3, 24E-3, 28E-3, 32E-3, 36E-3, 40E-3, 44E-3, 48E-3, 52E-3, 56E-3, 60E-3, 64E-3, 68E-3, 72E-3, 76E-3, 80E-3, 84E-3, 88E-3, 92E-3, 96E-3, 0.1, 96E-3, 92E-3, 88E-3, 84E-3, 80E-3, 76E-3, 72E-3, 68E-3, 64E-3, 60E-3, 56E-3, 52E-3, 48E-3, 44E-3, 40E-3, 36E-3, 32E-3, 28E-3, 24E-3, 20E-3, 16E-3, 12E-3, 8E-3, 4E-3, 0, -4E-3, -8E-3, -12E-3, -16E-3, -20E-3, -24E-3, -28E-3, -32E-3, -36E-3, -40E-3, -44E-3, -48E-3, -52E-3, -56E-3, -60E-3, -64E-3, -68E-3, -72E-3, -76E-3, -80E-3, -84E-3,\n            -88E-3, -92E-3, -96E-3, -0.1, -96E-3, -92E-3, -88E-3, -84E-3, -80E-3, -76E-3, -72E-3, -68E-3, -64E-3, -60E-3, -56E-3, -52E-3, -48E-3, -44E-3, -40E-3, -36E-3, -32E-3, -28E-3, -24E-3, -20E-3, -16E-3, -12E-3, -8E-3, -4E-3, 0, 4E-3, 8E-3, 12E-3, 16E-3, 20E-3, 24E-3, 28E-3, 32E-3, 36E-3, 40E-3, 44E-3, 48E-3, 52E-3, 56E-3, 60E-3, 64E-3, 68E-3, 72E-3, 76E-3, 80E-3, 84E-3, 88E-3, 92E-3, 96E-3, 0.1, 96E-3, 92E-3, 88E-3, 84E-3, 80E-3, 76E-3, 72E-3, 68E-3, 64E-3, 60E-3, 56E-3, 52E-3, 48E-3, 44E-3, 40E-3, 36E-3,\n        32E-3, 28E-3, 24E-3, 20E-3, 16E-3, 12E-3, 8E-3, 4E-3, 0, -4E-3, -8E-3, -12E-3, -16E-3, -20E-3, -24E-3, -28E-3, -32E-3, -36E-3, -40E-3, -44E-3, -48E-3, -52E-3, -56E-3, -60E-3, -64E-3, -68E-3, -72E-3, -76E-3, -80E-3, -84E-3, -88E-3, -92E-3, -96E-3, -0.1, -96E-3, -92E-3, -88E-3, -84E-3, -80E-3, -76E-3, -72E-3, -68E-3, -64E-3, -60E-3, -56E-3, -52E-3, -48E-3, -44E-3, -40E-3, -36E-3, -32E-3, -28E-3, -24E-3, -20E-3, -16E-3, -12E-3, -8E-3, -4E-3, 0" -> [_ w58]
    tunnel: [w46 w57] -> w8
    tunnel: "Source Code" -> [w45 w59]
    tunnel: w5 -> [w50 _]
    frame False {
      n10 = Number To Engineering String(2:i16 1 ("precision (6)"), 4:w50) -> (0:w54:string[])  [unwired: 2 in]
      n11 = call <vilib>:"1D String Array to Delimited String.vi"("delimiter"=",", "string array"=w54) -> ("delimited string"=w52:string)  [unwired: 9 in]
      n12 = Search and Replace String(input string=w45, search string="#VoltList", replace string=w52) -> (result string=w53:string)  [unwired: 5 in, 3 out]
      n13 = Array Size(array=w54) -> (size(s)=w55:i32)
      n14 = Number To Decimal String(number=w55) -> (decimal integer string=w56:string)  [unwired: 1 in]
      n15 = Search and Replace String(input string=w53, search string="#NumPoints", replace string=w56) -> (result string=w46:string)  [unwired: 5 in, 3 out]
    }
    frame True {
      n16 = Search and Replace String(input string=w59, search string="#VoltList", replace string=w58) -> (result string=w64:string)  [unwired: 5 in, 3 out]
      n17 = Number To Decimal String(number=200) -> (decimal integer string=w62:string)  [unwired: 1 in]
      n18 = Search and Replace String(input string=w64, search string="#NumPoints", replace string=w62) -> (result string=w57:string)  [unwired: 5 in, 3 out]
    }
  }
  n19 = while {
    tunnel: w29 -> [w81]
    tunnel: w30 -> [w80]
    tunnel: [w78] -> w28
    shift-right: [w72] -> w21
    shift-left: dbl[] [] ("array type (2D Dbl)") -> [w73]
    shift-right: [w70] -> w3
    shift-left: dbl[] [] ("array type (2D Dbl)") -> [w71]
    shift-right: [w77] -> w22
    shift-left: dbl[] [] ("array type (2D Dbl)") -> [w76]
    shift-right: [w75] -> w2
    shift-left: dbl[] [] ("array type (2D Dbl)") -> [w74]
    stop <- w65 stop-if-true
    w83 = 1 items=["Number", "Message"]  # Variable Type
    w82 = "Nil"  # Variable Name
    n20 = call "Print Variable.vi"("error in (no error)"=w80, "Variable Name"=w82, "Variable Type (0: Number)"=w83, "VISA resource name"=w81) -> ("error out"=→"error out":errorcluster, "Message"=w69:string, "VISA resource name out"=w78:refnum<visa-resource-name>)  [unwired: 4 in, 1 out]
    n21 = call <vilib>:"Trim Whitespace.vi"("string"=w69) -> ("trimmed string"=w68:string)  [unwired: 1 in]
    n22 = Not Equal?(x=w68, y="{COMPLETE}") -> (x != y?=w66:bool)
    n23 = Not(x=w66) -> (.not. x?=w65:bool)
    n24 = case shown="True" w66 {
      tunnel: w69 -> [_ w105]
      tunnel: [w87 w103] -> w77
      tunnel: w76 -> [w87 w102]
      tunnel: [w85 w100] -> w75
      tunnel: w74 -> [w85 w98]
      tunnel: w73 -> [w86 w97]
      tunnel: [w86 w96] -> w72
      tunnel: w71 -> [w84 w95]
      tunnel: [w84 w94] -> w70
      frame False {
      }
      frame True {
        # "Reads buffer data."
        n25 = Spreadsheet String To Array(delimiter (Tab)=",", format string="%.;%g", spreadsheet string=w105, array type (2D Dbl)=dbl[] []) -> (array=w91:dbl[])
        n26 = Array Size(array=w91) -> (size(s)=w90:i32)
        n27 = Index Array(array=w91, index=0) -> (element=w101:dbl)
        n28 = Subtract(x=w90, y=3) -> (x-y=w88:i32)
        n29 = To Long Integer(number=w101) -> (32bit integer=w99:i32)
        n30 = Array Subset(array=w91, index=2, length=w88) -> (w93:dbl[])
        n31 = case shown="2" w99 {
          tunnel: [w112 w120 w126 w132] -> w103
          tunnel: w102 -> [w114 w120 w126 w132]
          tunnel: [w111 w115 w125 w128] -> w100
          tunnel: w93 -> [w113 w118 w122 w130]
          tunnel: w98 -> [w111 w119 w125 w128]
          tunnel: w97 -> [w110 w117 w124 w131]
          tunnel: [w110 w117 w124 w129] -> w96
          tunnel: w95 -> [w109 w116 w123 w127]
          tunnel: [w109 w116 w121 w127] -> w94
          frame 0, Default {
            n32 = Build Array (concatenate)(w114, w113) -> (w112:dbl[])
          }
          frame 2 {
            n33 = Build Array (concatenate)(w119, w118) -> (w115:dbl[])
          }
          frame 3 {
            n34 = Build Array (concatenate)(w123, w122) -> (w121:dbl[])
          }
          frame 1 {
            n35 = Build Array (concatenate)(w131, w130) -> (w129:dbl[])
          }
        }
      }
    }
  }
  n36 = flat-sequence {
    tunnel: w1 -> [w133]
    frame #0 {
      w158 = 0.75 ("y")
      w175 = 5 ("y")
      w144 = T2 0 items=["Least Square", "Least Absolute Residual", "Bisquare"] ("method")
      n37 = Index Array(array=w133, index (row)=3) -> (element=w164:dbl[])  [unwired: 1 in]
      n38 = Index Array(array=w133, index (row)=2) -> (element=w165:dbl[])  [unwired: 1 in]
      n39 = Subtract(x=185, y=w175) -> (x-y=w176:i32)
      n40 = Array Subset(array=w165, index=w175, length=w176) -> (w156:dbl[])
      n41 = Array Max & Min(array=w156) -> (max value=w160:dbl, min value=w159:dbl)  [unwired: 2 out]
      n42 = Multiply(x=w160, y=w158) -> (x*y=w154:dbl)
      n43 = Multiply(x=w159, y=w158) -> (x*y=w153:dbl)
      n44 = Array Size(array=w156) -> (size(s)=w157:i32)
      n45 = Array Subset(array=w164, index=w175, length=w176) -> (w155:dbl[])
      n46 = for {
        N: w157 -> [_]
        tunnel: w156 -> [w211] mode=indexing
        tunnel: w155 -> [w210] mode=indexing
        tunnel: w154 -> [w215]
        tunnel: w153 -> [w214]
        shift-right: [w212] -> w149
        shift-left: _ -> [w213]
        shift-right: [w209] -> w150
        shift-left: _ -> [w208]
        n47 = Less?(x=w211, y=w215) -> (x < y?=w218:bool)
        n48 = Greater?(x=w211, y=w214) -> (0:w216:bool)
        n49 = And(x=w218, y=w216) -> (x .and. y?=w217:bool)
        n50 = case shown="True" w217 {
          tunnel: w213 -> [w220 w225]
          tunnel: [w220 w226] -> w212
          tunnel: w211 -> [_ w224]
          tunnel: w210 -> [_ w223]
          tunnel: [w219 w222] -> w209
          tunnel: w208 -> [w219 w221]
          frame False {
          }
          frame True {
            n51 = Build Array (concatenate)(w221, w223) -> (w222:dbl[])
            n52 = Build Array (concatenate)(w225, w224) -> (w226:dbl[])
          }
        }
      }
      n53 = Array Size(array=w149) -> (size(s)=w151:i32)
      n54 = for {
        N: w151 -> [_]
        tunnel: w149 -> [w185] mode=indexing
        tunnel: w150 -> [w182] mode=indexing
        shift-right: [w186] -> w146
        shift-left: _ -> [w187]
        shift-right: [w184] -> w145
        shift-left: _ -> [w183]
        shift-right: [w180] -> w148
        shift-left: _ -> [w177]
        shift-right: [w179] -> w147
        shift-left: _ -> [w178]
        n55 = Greater Than 0?(x=w182) -> (x > 0?=w181:bool)
        n56 = case shown="True" w181 {
          tunnel: w187 -> [w195 w202]
          tunnel: [w195 w203] -> w186
          tunnel: w185 -> [w189 w201]
          tunnel: w182 -> [w188 w200]
          tunnel: [w194 w199] -> w184
          tunnel: w183 -> [w194 w198]
          tunnel: [w193 w197] -> w180
          tunnel: [w192 w196] -> w179
          tunnel: w178 -> [w190 w196]
          tunnel: w177 -> [w191 w197]
          frame False {
            n57 = Build Array (concatenate)(w190, w188) -> (w192:dbl[])
            n58 = Build Array (concatenate)(w191, w189) -> (w193:dbl[])
          }
          frame True {
            n59 = Build Array (concatenate)(w202, w201) -> (w203:dbl[])
            n60 = Build Array (concatenate)(w198, w200) -> (w199:dbl[])
          }
        }
      }
      n61 = call <vilib>:"Linear Fit Coefficients.vi"("Y"=w147, "X"=w148, "method"=w144) -> ("slope"=w171:dbl, "intercept"=w172:dbl)  [unwired: 10 in, 1 out]
      n62 = call <vilib>:"Linear Fit Coefficients.vi"("Y"=w145, "X"=w146, "method"=w144) -> ("slope"=w143:dbl, "intercept"=w142:dbl)  [unwired: 10 in, 1 out]
      n63 = Build Array(w149, w150) -> (w161:dbl[][])
      n64 = Bundle(w149, w150) -> (w168:cluster{dbl[], dbl[]})  [unwired: 1 in]
      n65 = Build Array(w171, w172) -> (w163:dbl[])
      n66 = Build Array(w143, w142) -> (w140:dbl[])
      n67 = Add(x=w163, y=w140) -> (x+y=w141:dbl[])
      n68 = Divide(x=w141, y=2) -> (x/y=w138:dbl[])
      "Fit" <- w138
      n69 = case shown="True" FALSE {
        tunnel: w161 -> [_ w204]
        frame False {
        }
        frame True {
          n70 = call-poly <vilib>:"Write Delimited Spreadsheet.vi"("format (%.3f)"="%.9e", "2D data"=w204, "transpose? (no:F)"=TRUE, "delimiter (\\t)"="," ("delimiter (\\t)")) -> ()  [unwired: 10 in, 2 out]
        }
      }
      n71 = Index Array(array=w138, index=0) -> (element=w135:dbl)
      n72 = Index Array(array=w138, index=1) -> (element=w134:dbl)
      n73 = Multiply(x=w149, y=w135) -> (x*y=w173:dbl[])
      n74 = Add(x=w134, y=w173) -> (x+y=w174:dbl[])
      n75 = Bundle(w149, w174) -> (w169:cluster{dbl[], dbl[]})  [unwired: 1 in]
      n76 = Build Array(w168, w169) -> (→"XY Graph 2":cluster{dbl[], dbl[]}[])
    }
  }
  n77 = call "Close.vi"("error in (no error)"=w30, "VISA resource name"=w28) -> ("error out"=w31:errorcluster)  [unwired: 9 in]
  n78 = Build Array(w22, w21, w3, w2) -> (w1:dbl[][])
  "appended array" <- w1
  n79 = call <vilib>:"Simple Error Handler.vi"("error in (no error)"=w31) -> ()  [unwired: 4 in, 5 out]
  n80 = Bundle("array type (2D Dbl)"=w3, "array type (2D Dbl)"=w2) -> (→"Cluster" →"XY Graph":T1)  [unwired: 1 in]
  "Waveform Graph" <- "Waveform"
